vi "Read Error Count.vi"(11 "Method Result In":refnum<class "Method Result.lvclass">) -> (2 "Error count":i32, 3 "Method Result Out":refnum<class "Method Result.lvclass">)   [LabVIEW 2020, in "Method Result.lvclass"]
uses:
  Method Result.lvclass
  Assertion Result/Public/TypeDefs/Status.ctl
  Assertion Result/Assertion Result.lvclass
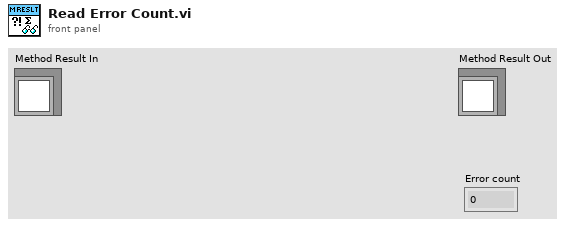
[diagram p1: front panel]
types:
  T1 = typedef "Assertion Result.lvclass/Status.ctl" = enum16{"Pass", "Fail", "Error", "Skipped", "Setup Error", "Broken", "Teardown Error"}
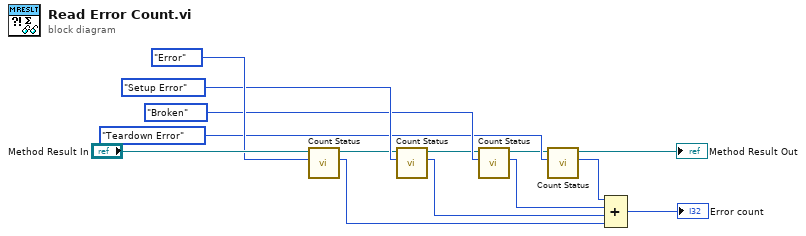
[diagram p0: block diagram]
diagram:
  n1 = call "Count Status.vi"("Status"=Status."Error", "Method Result in"="Method Result In") -> ("Count"=w3:i32, "Method Result out"=w9:refnum<class "Method Result.lvclass">)  [unwired: 8 in]
  n2 = call "Count Status.vi"("Status"=Status."Setup Error", "Method Result in"=w9) -> ("Count"=w4:i32, "Method Result out"=w8:refnum<class "Method Result.lvclass">)  [unwired: 8 in]
  n3 = call "Count Status.vi"("Status"=Status."Broken", "Method Result in"=w8) -> ("Count"=w5:i32, "Method Result out"=w7:refnum<class "Method Result.lvclass">)  [unwired: 8 in]
  n4 = call "Count Status.vi"("Status"=Status."Teardown Error", "Method Result in"=w7) -> ("Count"=w6:i32, "Method Result out"=→"Method Result Out":refnum<class "Method Result.lvclass">)  [unwired: 8 in]
  n5 = Compound Arithmetic op=ADD(w6, w5, w4, w3) -> (→"Error count":i32)
